vi "Add Virtual Instruments.vi"(6 "<JSON CFG>":string, 8 "error in":errorcluster, 11 "Host Measure and Stimulus Subsystems in":refnum<class "Host Measure and Stimulus Subsystems.lvclass">) -> (0 "error out":errorcluster, 3 "Host Measure and Stimulus Subsystems out":refnum<class "Host Measure and Stimulus Subsystems.lvclass">)   [LabVIEW 2023, in "HAL GOOP4.lvlib" / "Host Measure and Stimulus Subsystems.lvclass"]
uses:
  Host Measure and Stimulus Subsystems.lvclass
  90214a18-2aad-49f1-98b3-b69aa3edef87.vi
  <vilib>/JDP Science/JSONtext/Find Item.vi
  <vilib>/JDP Science/JSONtext/Next JSON Value.vi
  <vilib>/JDP Science/JSONtext/String Subset.vi
  <vilib>/JDP Science/JSONtext/Parsing/Advance past next JSON Value (inlined COPY).vi
  <vilib>/JDP Science/JSONtext/Parsing/Advance past whitespace.vi
  <vilib>/JDP Science/JSONtext/Parsing/Advance past String.vi
  <vilib>/JDP Science/JSONtext/Parsing/Advance past Number.vi
  <vilib>/JDP Science/JSONtext/Parsing/Advance past Line Ending.vi
  <vilib>/JDP Science/JSONtext/Parsing/Parse Full Path or Item Name.vi
  <vilib>/JDP Science/JSONtext/Parsing/Advance past Array.vi
  <vilib>/JDP Science/JSONtext/Parsing/Advance past Object.vi
  <vilib>/JDP Science/JSONtext/support/Error Cluster From Code.vi
  <vilib>/JDP Science/JSONtext/Offset/Find Item Locations by Path.vi
  <vilib>/JDP Science/JSONtext/JSON text to Variant.vi
  <vilib>/Utility/error.llb/Error Cluster From Error Code.vi
  <vilib>/JDP Science/JSONtext/LVClass Serializer/JSONtext LVClass Serializer.lvclass
  <vilib>/ErrorRing/Error Ring.xnode
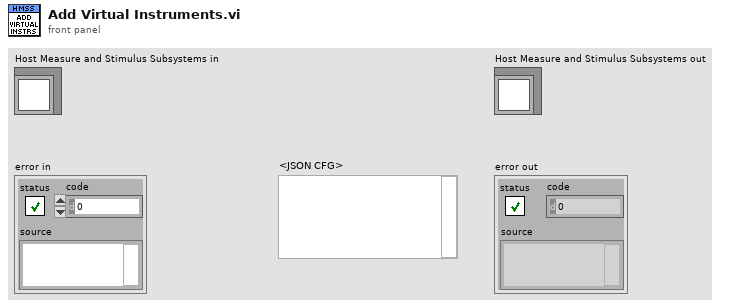
[diagram p1: front panel]
types:
  T1 = cluster{"Target Ident":string, "Instr Ident":string, "Const Action Data":string, "Class":string}[]
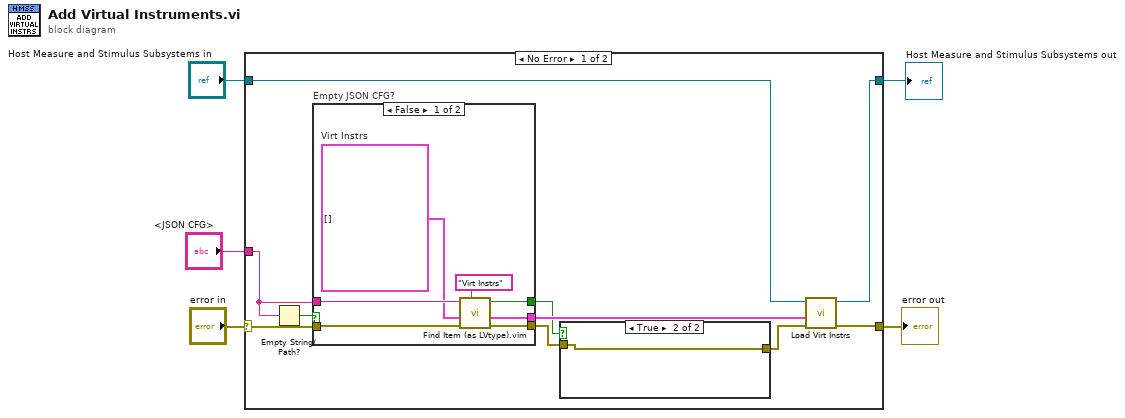
[diagram p0: block diagram]
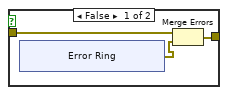
[diagram p2: hidden frame]
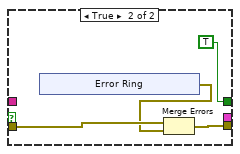
[diagram p3: hidden frame]
diagram:
  n1 = case shown="No Error" "error in" {
    selector: "error in" -> [w13 w42]
    tunnel: [w15 w42] -> w1
    tunnel: [w6 w41] -> w2
    tunnel: "Host Measure and Stimulus Subsystems in" -> [w7 w41]
    tunnel: "<JSON CFG>" -> [w11 _]
    frame No Error {
      n2 = Empty String/Path?(string/path=w11) -> (empty?=w12:bool)
      n3 = case "Empty JSON CFG?" shown="False" w12 {
        tunnel: w13 -> [w31 w35]
        tunnel: [w29 w33] -> w8
        tunnel: w11 -> [w30 _]
        tunnel: [w26 _] -> w14
        tunnel: [w25 TRUE ("Found")] -> w9
        frame False {
          w28 = T1 []  # Virt Instrs
          n4 = call "Find Item (as LVtype).vim"("$Path or Item Name"="Virt Instrs", "error in (no error)"=w31, "Data Type and Default Value"=w28, "JSON"=w30) -> ("error out"=w29:errorcluster, "Data"=w26:T1, "Found"=w25:bool)  [unwired: 4 in, 1 out]
        }
        frame True {
          n5 = xnode "Error Ring"() -> ("error out"=w34:errorcluster)
          n6 = Merge Errors(w35, w34) -> (w33:errorcluster)
        }
      }
      n7 = case shown="True" w9 {
        tunnel: [w18 w24] -> w10
        tunnel: w8 -> [w16 w24]
        frame False {
          n8 = xnode "Error Ring"() -> ("error out"=w17:errorcluster)
          n9 = Merge Errors(w16, w17) -> (w18:errorcluster)
        }
        frame True {
        }
      }
      n10 = call-dynamic "Load Virt Instrs.vi"("error in"=w10, "JSON Virt Instrs"=w14, "Host Measure and Stimulus Subsystems in"=w7) -> ("error out"=w15:errorcluster, "Host Measure and Stimulus Subsystems out"=w6:refnum<class "Host Measure and Stimulus Subsystems.lvclass">)  [unwired: 7 in]
    }
    frame Error {
    }
  }
  "error out" <- w1
  "Host Measure and Stimulus Subsystems out" <- w2
